vi "swabian_chart_counts.vi"(8 "error in (no error)":errorcluster, 11 "swabian_local_data":T1={"events"={"update_status"=refnum, "update_chart"=refnum, "update_xy"=refnum, "send_channel_data"=refnum}, "stop_q"=refnum, "tagger_reference"=refnum, "connect_button"=refnum, "counter_reference"=refnum, "tagger_stream_reference"=refnum, "log_reference"=refnum, "current_log_offset"=0, "tt20_buffer_q"=refnum, "stream_to_file_button"=refnum, "num_records"=0, "connected?"=FALSE, "plots"=refnum, "histogram_bin_edges"=[], "histogrammer"=refnum, "plot_lifetimes"=refnum, "xy_graph"=refnum, "Reference\nChannel"=enum."ch0", "trigger_channels"=[], "filter_channels"=[], "active_channels"=[], "acq_mode"=0, "Reference\nChannel"=enum."ch0", "acq_time"=0, "sync_period_ps"=0, "raw_stream_path"=path "", "Leftovers"={"missing_sync_data"=[], "missing_events"=0}, "first_batch"=0, "first_sync_stamp"=0, "lifetime_settings"={"Plot Lifetimes"=FALSE, "start_time"=0.0, "stop_time"=0.0, "n_bins"=0, "Oscilloscope"=TRUE}, "Histogram_bins"=[], "last_processed_data"=[], "histogram_data"=[]}) -> (0 "error IO":errorcluster, 3 "swabian_local_data 2":T1={"events"={"update_status"=refnum, "update_chart"=refnum, "update_xy"=refnum, "send_channel_data"=refnum}, "stop_q"=refnum, "tagger_reference"=refnum, "connect_button"=refnum, "counter_reference"=refnum, "tagger_stream_reference"=refnum, "log_reference"=refnum, "current_log_offset"=0, "tt20_buffer_q"=refnum, "stream_to_file_button"=refnum, "num_records"=0, "connected?"=FALSE, "plots"=refnum, "histogram_bin_edges"=[], "histogrammer"=refnum, "plot_lifetimes"=refnum, "xy_graph"=refnum, "Reference\nChannel"=enum."ch0", "trigger_channels"=[], "filter_channels"=[], "active_channels"=[], "acq_mode"=0, "Reference\nChannel"=enum."ch0", "acq_time"=0, "sync_period_ps"=0, "raw_stream_path"=path "", "Leftovers"={"missing_sync_data"=[], "missing_events"=0}, "first_batch"=0, "first_sync_stamp"=0, "lifetime_settings"={"Plot Lifetimes"=FALSE, "start_time"=0.0, "stop_time"=0.0, "n_bins"=0, "Oscilloscope"=TRUE}, "Histogram_bins"=[], "last_processed_data"=[], "histogram_data"=[]})   [LabVIEW 2018]
uses:
  swabian_local_data_tdef.ctl
  swabian_events_tdef.ctl
  update_chart_tdef.ctl
  channel_data_tdef.ctl
  C:/Users/bspoka/Documents/swabian_LV/lib/TTCSharp32.dll
  lib/TTCSharp32.dll
  swabian_buffer_tdef.ctl
  reference_checkbox_tdef.ctl
  lifetime_settings.ctl
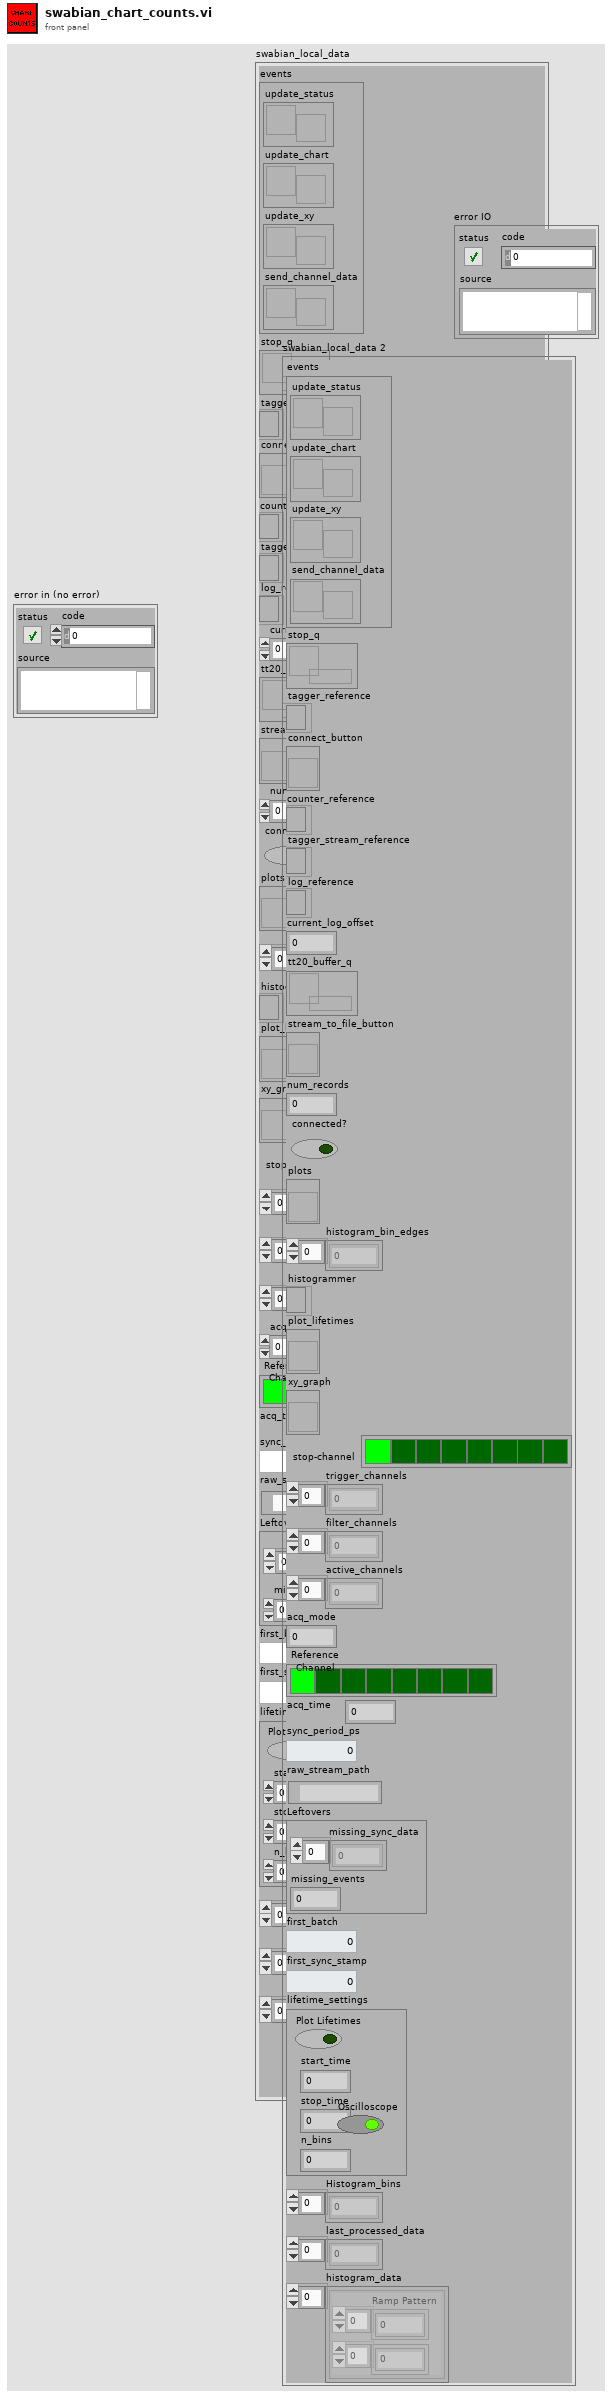
[diagram p1: front panel]
types:
  T1 = typedef "swabian_local_data_tdef.ctl" = cluster{"events":T2, "stop_q":refnum<queue>, "tagger_reference":refnum<k24>, "connect_button":refnum<vi>, "counter_reference":refnum<k24>, "tagger_stream_reference":refnum<k24>, "log_reference":refnum<file>, "current_log_offset":i64, "tt20_buffer_q":refnum<queue>, "stream_to_file_button":refnum<vi>, "num_records":u64, "connected?":bool, "plots":refnum<vi>, "histogram_bin_edges":i64[], "histogrammer":refnum<k24>, "plot_lifetimes":refnum<vi>, "xy_graph":refnum<vi>, "Reference\nChannel":T3, "trigger_channels":i32[], "filter_channels":i32[], "active_channels":i32[], "acq_mode":i32, "Reference\nChannel":T3, "acq_time":i64, "sync_period_ps":i64, "raw_stream_path":path, "Leftovers":cluster{"missing_sync_data":i64[], "missing_events":i32}, "first_batch":i32, "first_sync_stamp":i64, "lifetime_settings":T4, "Histogram_bins":dbl[], "last_processed_data":i64[], "histogram_data":cluster{"Ramp Pattern":dbl[], dbl[]}[]}
  T2 = typedef "swabian_events_tdef.ctl" = cluster{"update_status":refnum<user-event>, "update_chart":refnum<user-event>, "update_xy":refnum<user-event>, "send_channel_data":refnum<user-event>}
  T3 = typedef "reference_checkbox_tdef.ctl" = enum32{"No Selection", "ch0", "ch1", "ch2", "ch3", "ch4", "ch5", "ch6", "ch7"}
  T4 = typedef "lifetime_settings.ctl" = cluster{"Plot Lifetimes":bool, "start_time":dbl, "stop_time":dbl, "n_bins":i32, "Oscilloscope":bool}
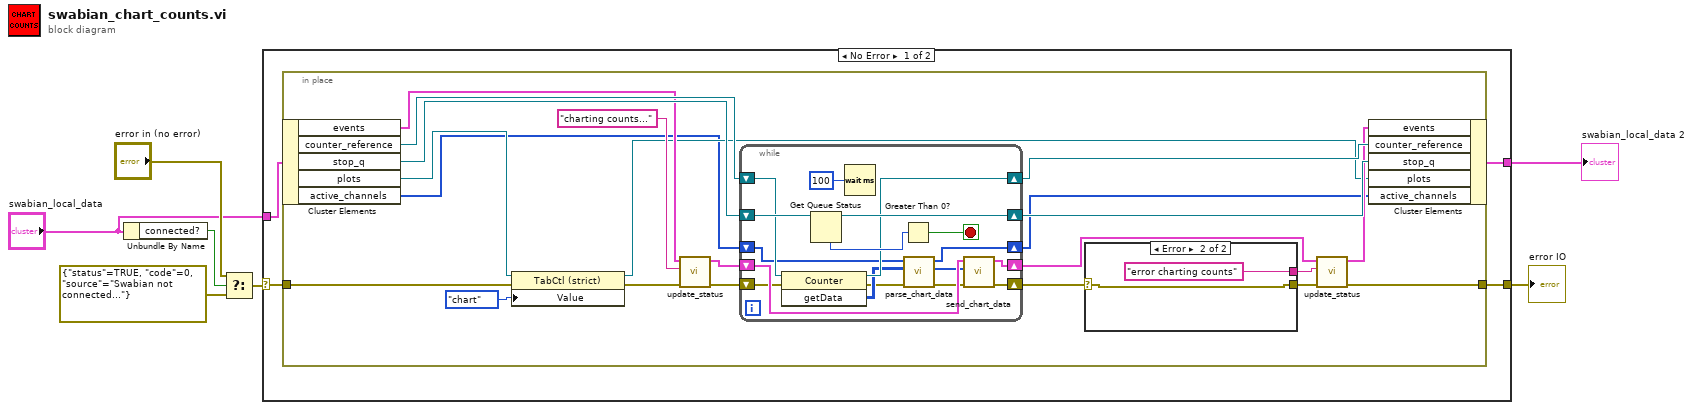
[diagram p0: block diagram]
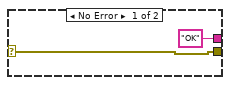
[diagram p2: hidden frame]
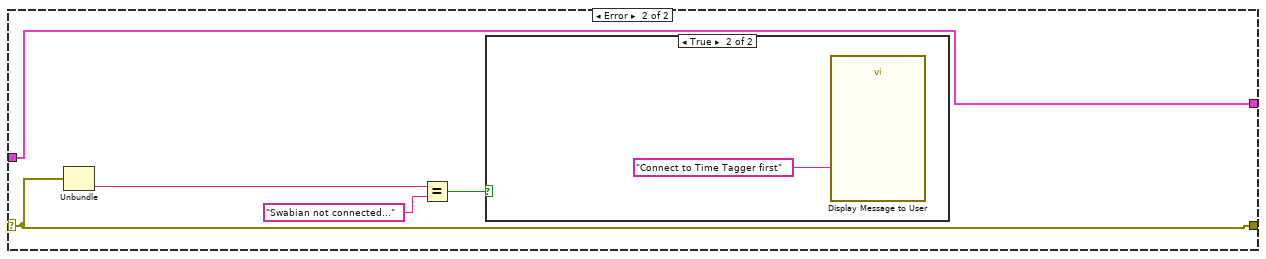
[diagram p3: hidden frame]
diagram:
  n1 = Unbundle By Name("swabian_local_data") -> ("connected?"=w5:bool)
  n2 = Select(t="error in (no error)", s=w5, f=errorcluster {"status"=TRUE, "code"=0, "source"="Swabian not connected..."}) -> (s? t:f=w2:errorcluster)
  n3 = case shown="No Error" w2 {
    selector: w2 -> [w11 w55]
    tunnel: [w8 w55] -> w7
    tunnel: "swabian_local_data" -> [w10 w58]
    tunnel: [w9 w58] -> w6
    frame No Error {
      n4 = in-place {
        in-place-border: w11 -> [w18]
        in-place-border: [w22] -> w8
        n5 = in-place-cluster #1(w10) -> ("events"=w27:T2, "counter_reference"=w32:refnum<k24>, "stop_q"=w31:refnum<queue>, "plots"=w16:refnum<vi>, "active_channels"=w13:i32[])
        n6 = property class="TabCtl (strict)"(reference=w16, error in=w18, "Value"=enum32{"chart", "xy_graph"}."chart") -> (reference out=w15:refnum<vi>, error out=w17:errorcluster)
        n7 = call "update_status.vi"("error in (no error)"=w17, "status"="charting counts...", "events"=w27) -> ("error out"=w28:errorcluster, "events_out"=w26:T2)  [unwired: 7 in]
        n8 = while {
          shift-right: [w47] -> w24
          shift-left: w28 -> [w44]
          shift-right: [w48] -> w20
          shift-left: w26 -> [w49]
          shift-right: [w43] -> w30
          shift-left: w32 -> [w45]
          shift-right: [w46] -> w29
          shift-left: w31 -> [w52]
          shift-right: [w40] -> w12
          shift-left: w13 -> [w41]
          stop <- w50 stop-if-true
          n9 = invoke class="Counter" method="getData"(reference=w45, error in=w44) -> (reference out=w43:refnum<k24>, error out=w37:errorcluster, "getData"=w42:i32[][])  [unwired: 1 in]
          n10 = Get Queue Status(queue=w52) -> (queue out=w46:refnum<queue>, # elements in queue=w51:i32)  [unwired: 2 in, 6 out]
          n11 = Wait (ms)(milliseconds to wait=u32 100) -> ()  [unwired: 1 out]
          n12 = Greater Than 0?(x=w51) -> (x > 0?=w50:bool)
          n13 = call "parse_chart_data.vi"("error constant"=w37, "swabian_data_in"=w42, "active_channels"=w41) -> ("error constant 2"=w38:errorcluster, "formatted_data"=w39:i32[], "active_channels_out"=w40:i32[])  [unwired: 6 in]
          n14 = call "send_chart_data.vi"("error in (no error)"=w38, "getData"=w39, "events"=w49) -> ("error in (no error) 2"=w47:errorcluster, "events 2"=w48:T2)  [unwired: 7 in]
        }
        n15 = case shown="Error" w24 {
          selector: w24 -> [w34 w35]
          tunnel: [w34 w35] -> w23
          tunnel: ["OK" ("status") "error charting counts" ("status")] -> w19
          frame No Error {
          }
          frame Error {
          }
        }
        n16 = call "update_status.vi"("error in (no error)"=w23, "status"=w19, "events"=w20) -> ("error out"=w22:errorcluster, "events_out"=w21:T2)  [unwired: 7 in]
        n17 = in-place-cluster #1("events"=w21, "counter_reference"=w30, "stop_q"=w29, "plots"=w15, "active_channels"=w12) -> (w9:T1)
      }
    }
    frame Error {
      n18 = Unbundle(w55) -> ("source"=w57:string)  [unwired: 2 out]
      n19 = Equal?(x=w57, y="Swabian not connected..." ("source")) -> (x = y?=w54:bool)
      n20 = case shown="True" w54 {
        frame False {
        }
        frame True {
          n21 = call "Display Message to User"("Message"="Connect to Time Tagger first") -> ()  [unwired: 9 in, 2 out]
        }
      }
    }
  }
  "error IO" <- w7
  "swabian_local_data 2" <- w6
